vi "PH_SSAC.Draw Image.vi"(0 "i ref in":refnum<vi>, 2 "Image":T1, 5 "error in (no error)":errorcluster) -> (14 "i ref out":refnum<vi>, 17 "Status":T2 items=["no info", "off/false/out", "on/true/in", "Failure", "Alarm", "Status 1", "Status 2", "Status 3"], 19 "error out":errorcluster)   [LabVIEW 2014, in "PH_SSAC.lvlib"]
doc: "This VI draws the image to the GUI. Depending on the sequencer state, it writes the images also to the attributes or calculates the pixel sum."
uses:
  PH_SSAC.lvlib
  PH_StatusHandler/PH_StatusHandler.Status.ctl
  <vilib>/vision/Image Controls.llb/IMAQ Image.ctl
  PH_StatusHandler/PH_StatusHandler.lvlib
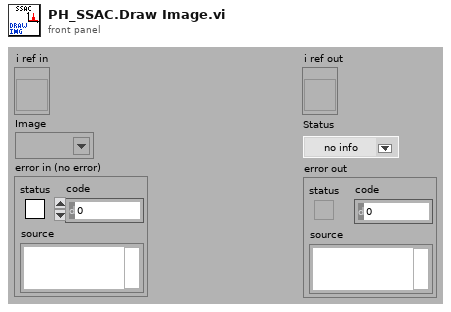
[diagram p1: front panel]
types:
  T1 = typedef "IMAQ Image.ctl" = refnum<image>
  T2 = typedef "PH_StatusHandler.lvlib/PH_StatusHandler.Status.ctl" = i16
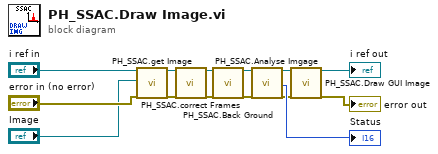
[diagram p0: block diagram]
diagram:
  n1 = call "PH_SSAC.get Image.vi"("i ref in"="i ref in", "Image (dup)"="Image", "error in (no error)"="error in (no error)") -> ("i ref out"=w8:refnum<vi>, "error out"=w7:errorcluster)  [unwired: 15 in]
  n2 = call "PH_SSAC.correct Frames.vi"("i ref in"=w8, "error in"=w7) -> ("i ref out"=w6:refnum<vi>, "error out"=w5:errorcluster)  [unwired: 16 in]
  n3 = call "PH_SSAC.Back Ground.vi"("i ref in"=w6, "error in"=w5) -> ("i ref out"=w2:refnum<vi>, "error out"=w4:errorcluster)  [unwired: 16 in]
  n4 = call "PH_SSAC.Analyse Imgage.vi"("i ref in"=w2, "error in"=w4) -> ("i ref out"=w1:refnum<vi>, "Status"=→"Status":T2, "error out"=w3:errorcluster)  [unwired: 15 in]
  n5 = call "PH_SSAC.Draw GUI Image.vi"("i ref in"=w1, "error in"=w3) -> ("i ref out"=→"i ref out":refnum<vi>, "error out"=→"error out":errorcluster)  [unwired: 16 in]
